vi "DeleteAction.vi"(8 "Error In":errorcluster, 9 "Analysis List":refnum<vi>, 10 "Analysis Step":i32[](listbox), 11 "CoordinatteEntry In":T1={"ProcessSetting"=[], "Project Name"="Parttern", "AnalysisSetting"=[], "Coord?"=FALSE, "OriginPointInfo"={"Output Original"=FALSE, "Origin Name"="", "Angle"=0.0, "Mode"=0, "OriginPoint"={"X"=0.0, "Y"=0.0}}, "CaliperSetting"=[], "CoordIndex"=[]} {"CaliperSetting"."CaliperEntry"."CaliperType" items=["Distance", "Mid Point", "Perpendicular Projection", "Lines Intersection", "Angle from Horizontal", "Angle from Vertical", "Angle Defined by 3 Points", "Angle Defined by 4 Points", "Bissecting Line", "Mid Line", "Center of Mass", "Area", "Line Fit", "Circle Fit", "Ellipse Fit"]; "OriginPointInfo"."Mode" items=["Horizontal Motion", "Vertical Motion", "Horizontal and Vertical Motion", "Horizontal. Vertical and Angular Motion"]; "AnalysisSetting"."ROI"."Contours"."Type" items=["No Selection", "Point", "Line", "Rectangle", "Oval", "Polygon", "Freehand Region", "Annulus", "Unused2", "Unused3", "Broken Line", "Freehand Line", "Rotated Rectangle"]}) -> (0 "Error Out":errorcluster, 3 "CoordinatteEntry Out":T1={"ProcessSetting"=[], "Project Name"="Parttern", "AnalysisSetting"=[], "Coord?"=FALSE, "OriginPointInfo"={"Output Original"=FALSE, "Origin Name"="", "Angle"=0.0, "Mode"=0, "OriginPoint"={"X"=0.0, "Y"=0.0}}, "CaliperSetting"=[], "CoordIndex"=[]} {"CaliperSetting"."CaliperEntry"."CaliperType" items=["Distance", "Mid Point", "Perpendicular Projection", "Lines Intersection", "Angle from Horizontal", "Angle from Vertical", "Angle Defined by 3 Points", "Angle Defined by 4 Points", "Bissecting Line", "Mid Line", "Center of Mass", "Area", "Line Fit", "Circle Fit", "Ellipse Fit"]; "OriginPointInfo"."Mode" items=["Horizontal Motion", "Vertical Motion", "Horizontal and Vertical Motion", "Horizontal. Vertical and Angular Motion"]; "AnalysisSetting"."ROI"."Contours"."Type" items=["No Selection", "Point", "Line", "Rectangle", "Oval", "Polygon", "Freehand Region", "Annulus", "Unused2", "Unused3", "Broken Line", "Freehand Line", "Rotated Rectangle"]})   [LabVIEW 2015]
uses:
  Control/CoordinatteEntry.ctl
  Process/Controls/Process_Setting.ctl
  Process/Controls/Process_Type.ctl
  Control/CoordinateAnalysisSetting.ctl
  Control/CoordinateCaliperSetting.ctl
  Caliper/Controls/CaliperDataEntry.ctl
  Caliper/Controls/CaliperType.ctl
  Caliper/Controls/SelectionListEntry.ctl
  Caliper/Controls/SelectionListEntryPointType.ctl
  Caliper/Controls/CaliperResult.ctl
  Analysis/Controls/Parttern Match/Analysis_PatternMatch_Parameter.ctl
panel:
  out "RootPath":path
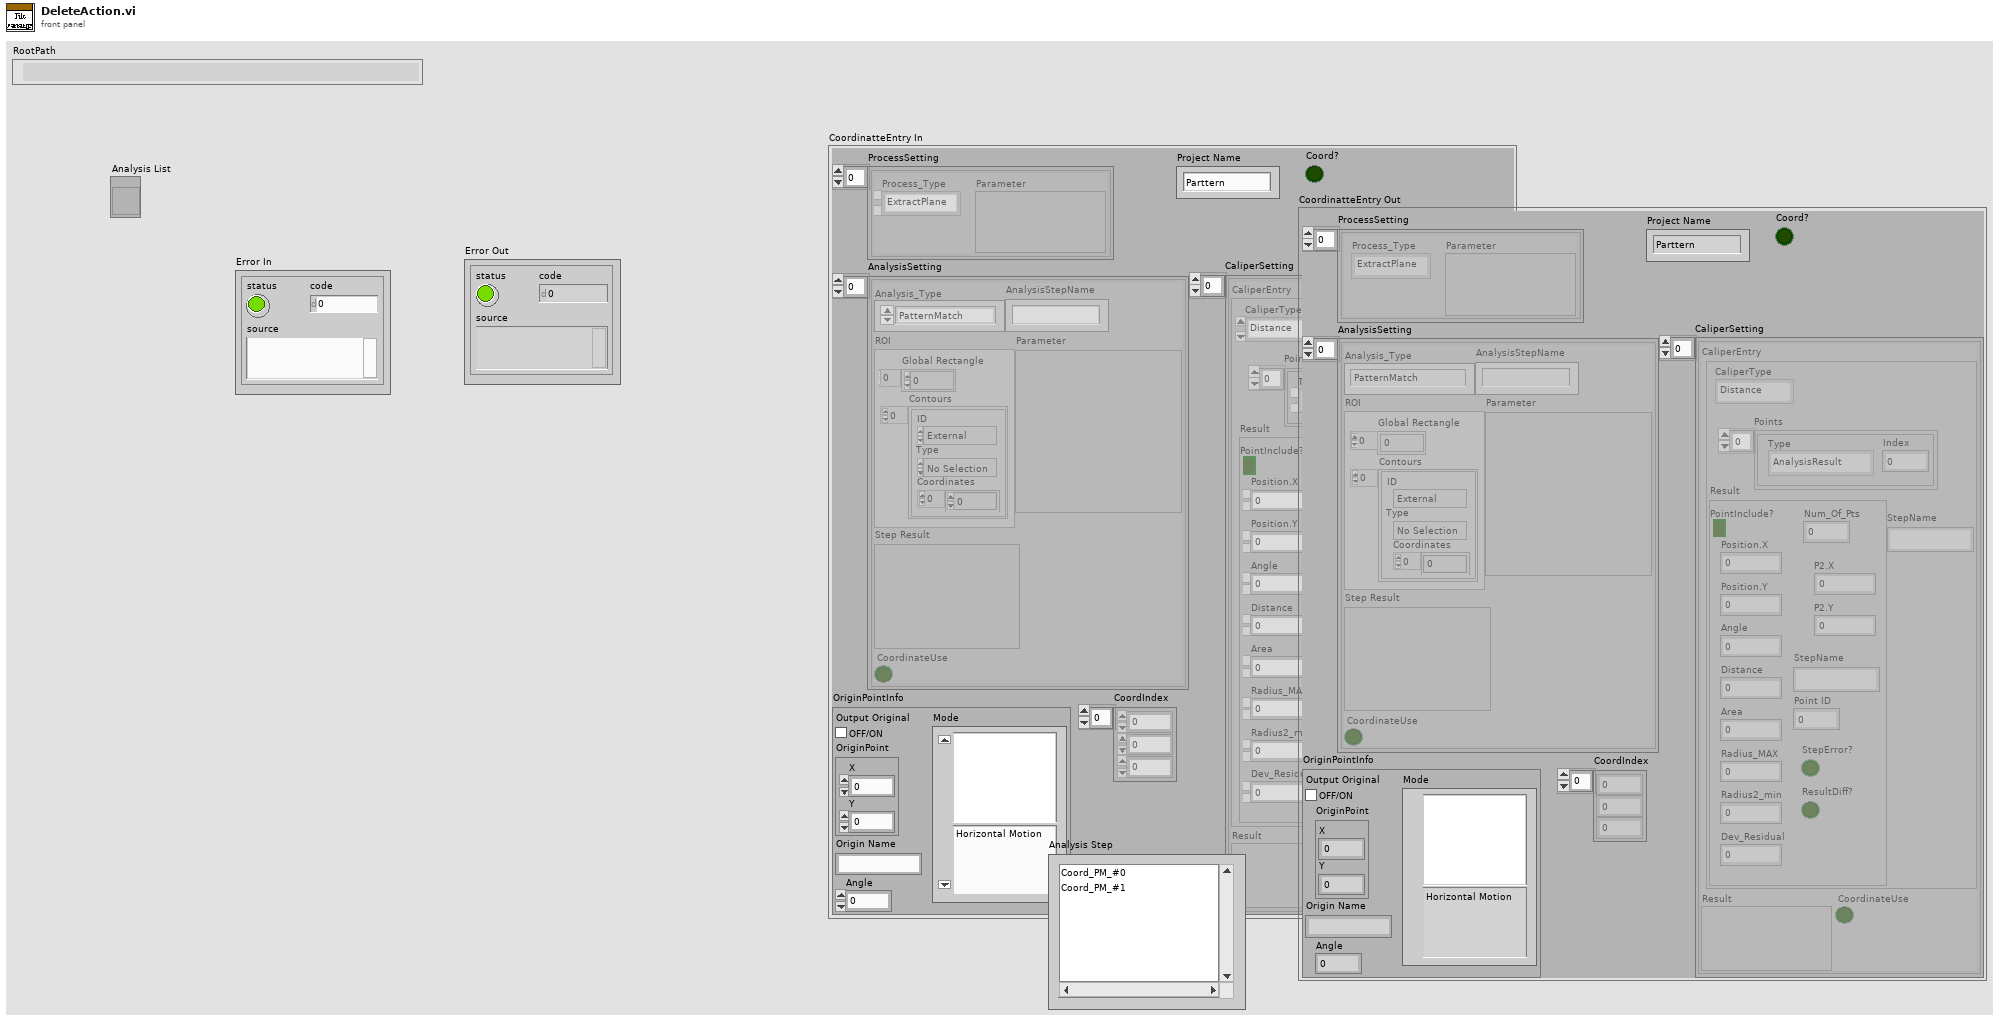
[diagram p1: front panel]
types:
  T1 = typedef "CoordinatteEntry.ctl" = cluster{"ProcessSetting":T2[], "Project Name":string, "AnalysisSetting":T4[], "Coord?":bool, "OriginPointInfo":cluster{"Output Original":bool, "Origin Name":string, "Angle":dbl, "Mode":u16, "OriginPoint":cluster{"X":dbl, "Y":dbl}}, "CaliperSetting":T6[], "CoordIndex":i32[]}
  T2 = typedef "Process_Setting.ctl" = cluster{"Process_Type":T3, "Parameter":variant}
  T3 = typedef "Process_Type.ctl" = enum16{"None", "ExtractPlane", "BinaryMono", "Operators", "GrayMorphology", "Filters", "Lookup Table", "Particle Filter", "Mask"}
  T4 = typedef "CoordinateAnalysisSetting.ctl" = cluster{"Analysis_Type":enum16{"PatternMatch", "Straight Edge"}, "ROI ":T5, "Parameter":variant, "Step Result":variant, "AnalysisStepName":string, "CoordinateUse":bool}
  T5 = typedef "ROI Descriptor" = cluster{"Global Rectangle":i32[], "Contours":cluster{"ID":enum32{"External", "Internal"}, "Type":u32, "Coordinates":i32[]}[]}
  T6 = typedef "CoordinateCaliperSetting.ctl" = cluster{"Result":variant, "CoordinateUse":bool, "CaliperEntry":T7}
  T7 = typedef "CaliperDataEntry.ctl" = cluster{"CaliperType":T8, "Points":T9[], "Result":T11, "StepName":string}
  T8 = typedef "CaliperType.ctl" = u32
  T9 = typedef "SelectionListEntry.ctl" = cluster{"Type":T10, "Index":i32}
  T10 = typedef "SelectionListEntryPointType.ctl" = enum16{"AnalysisResult", "CaliperResult"}
  T11 = typedef "CaliperResult.ctl" = cluster{"PointInclude?":bool, "Num_Of_Pts":u8, "Position.X":dbl, "Position.Y":dbl, "Angle":dbl, "Distance":dbl, "Area":dbl, "Radius_MAX":dbl, "Radius2_min":dbl, "Dev_Residual":dbl, "P2.X":dbl, "P2.Y":dbl, "StepName":string, "Point ID":u8, "StepError?":bool, "ResultDiff?":bool}
  T12 = enum32{"invalid app kind", "Development System", "Run Time System", "Student Edition", "Embedded LabVIEW", "Evaluation", "Custom"}
  T13 = typedef "Analysis_PatternMatch_Parameter.ctl" = cluster{"Algorithm":i32, "Match Parameters":cluster{"Number of Matches Requested":i32, "Minimum Match Score":sgl, "Angle Ranges":cluster{"Start Angle":sgl, "End Angle":sgl}[]}, "ROI Descriptor":T5, "Advanced Options":cluster{"Item":u16, "Value":dbl}[], "Template path":string, "XOffset":i32, "YOffset":i32}
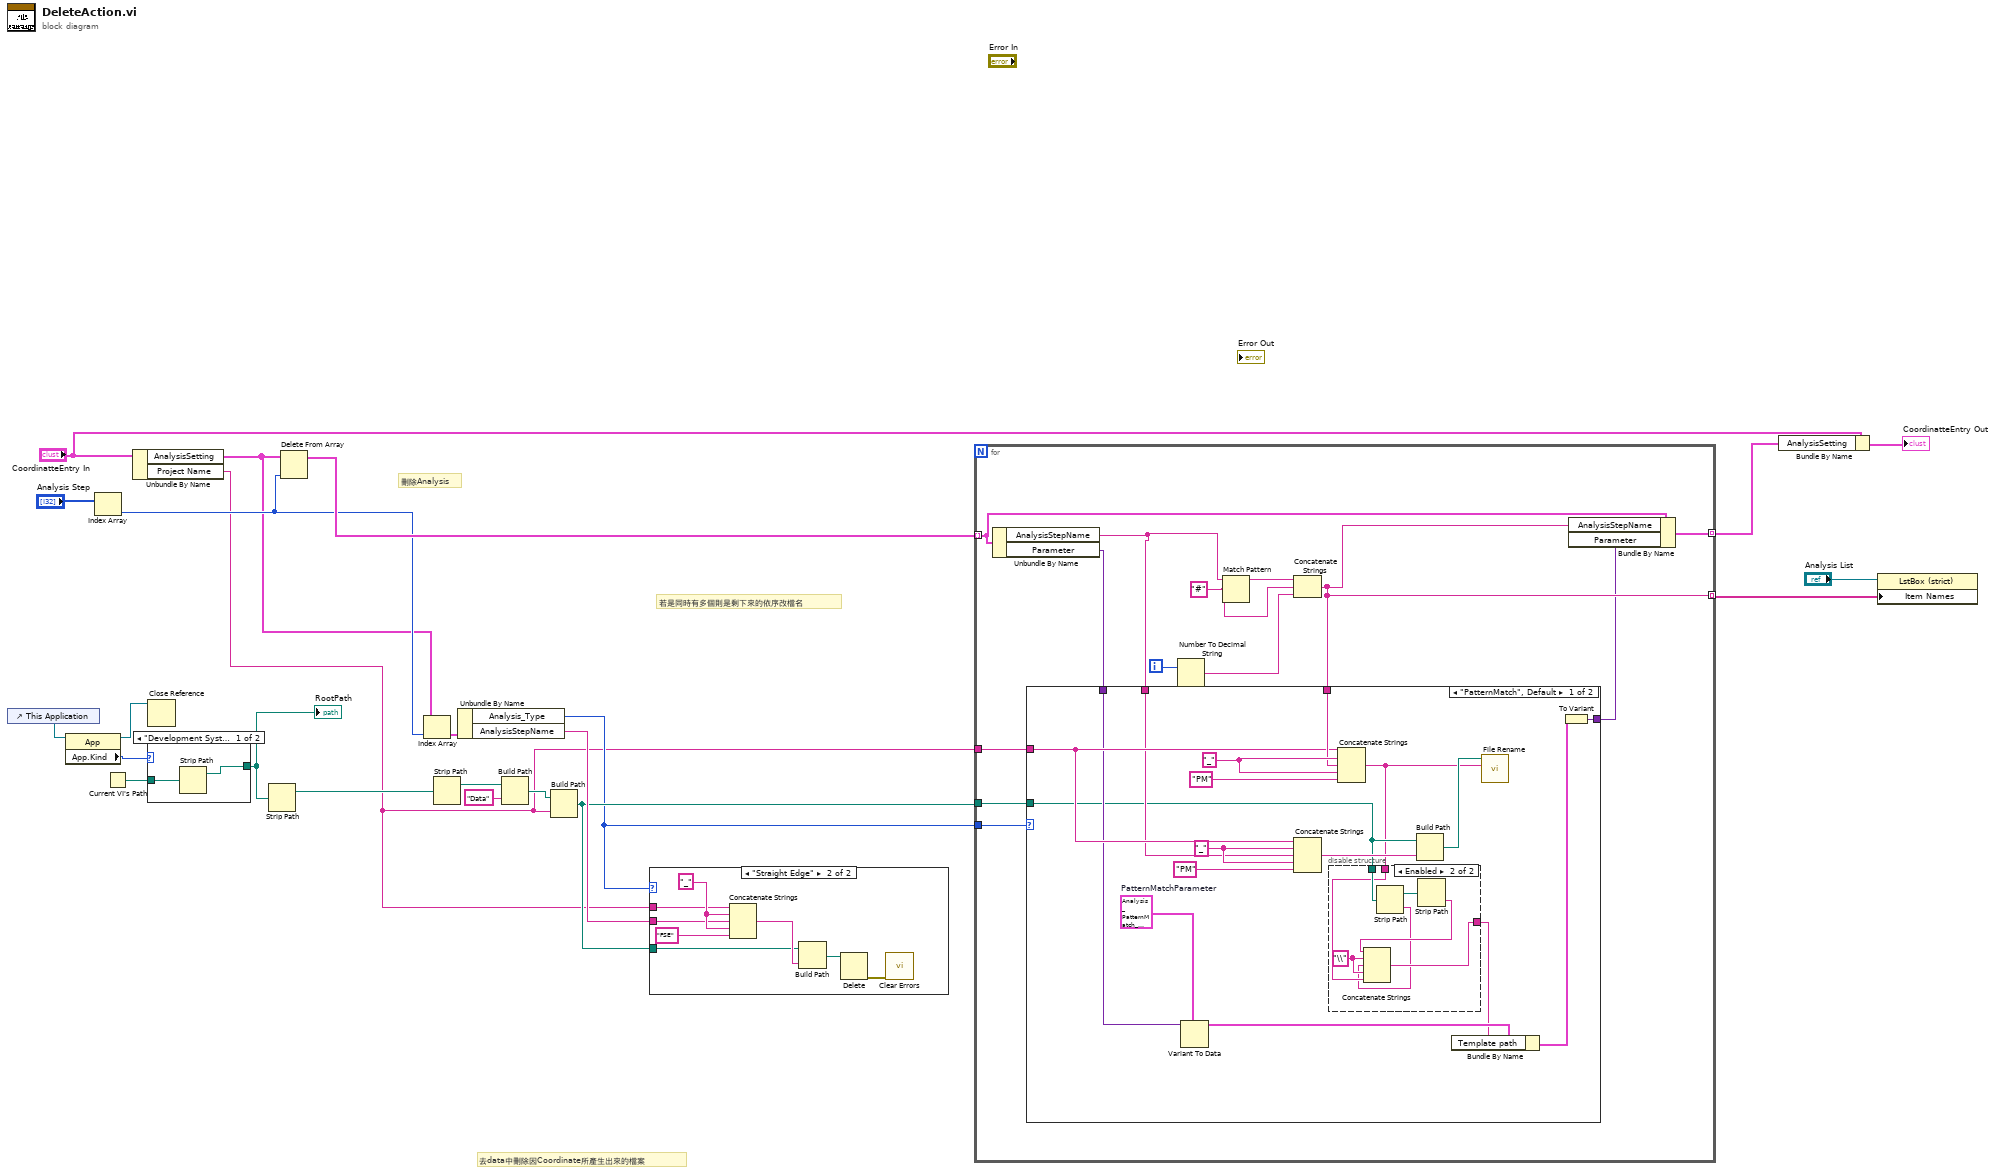
[diagram p0: block diagram]
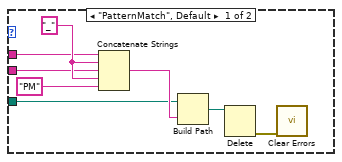
[diagram p2: hidden frame]
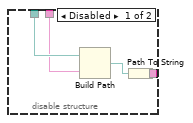
[diagram p3: hidden frame]
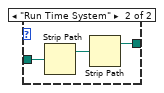
[diagram p5: hidden frame]
diagram:
  # "若是同時有多個則是剩下來的依序改檔名"
  # "去data中刪除因Coordinate所產生出來的檔案"
  # "刪除Analysis"
  n1 = control-ref of="This Application"() -> (w20:refnum<vi>)
  n2 = property class="App"(reference=w20) -> (reference out=w22:refnum<vi>, "App.Kind"=w21:T12)  [unwired: 1 in, 1 out]
  n3 = Index Array(array="Analysis Step") -> (element=w8:i32)  [unwired: 1 in]
  n4 = Current VI's Path() -> (path=w23:path)
  n5 = Unbundle By Name("CoordinatteEntry In") -> ("AnalysisSetting"=w6:T4[], "Project Name"=w1:string)
  n6 = case shown="\"Development System\", Default" w21 {
    tunnel: w23 -> [w25 w28]
    tunnel: [w24 w26] -> w19
    frame "Development System", Default {
      n7 = Strip Path(path=w25) -> (stripped path=w24:path)  [unwired: 1 out]
    }
    frame "Run Time System" {
      n8 = Strip Path(path=w28) -> (stripped path=w27:path)  [unwired: 1 out]
      n9 = Strip Path(path=w27) -> (stripped path=w26:path)  [unwired: 1 out]
    }
  }
  "RootPath" <- w19
  n10 = Close Reference(reference=w22) -> ()  [unwired: 1 in, 1 out]
  n11 = Strip Path(path=w19) -> (stripped path=w18:path)  [unwired: 1 out]
  n12 = Delete From Array "Delete From Array"(array=w6, index=w8) -> (array with subset deleted=w14:T4[])  [unwired: 1 in, 1 out]
  n13 = Index Array(array=w6, index=w8) -> (element=w7:T4)
  n14 = Strip Path(path=w18) -> (stripped path=w17:path)  [unwired: 1 out]
  n15 = Unbundle By Name(w7) -> ("Analysis_Type"=w2:enum16{"PatternMatch", "Straight Edge"}, "AnalysisStepName"=w4:string)
  n16 = Build Path(base path=w17, name or relative path="Data") -> (appended path=w15:path)
  n17 = Build Path(base path=w15, name or relative path=w1) -> (appended path=w3:path)
  n18 = case shown="\"Straight Edge\"" w2 {
    tunnel: w1 -> [w31 w39]
    tunnel: w4 -> [w30 w38]
    tunnel: w3 -> [w29 w37]
    frame "PatternMatch", Default {
      w35 = "_" ("string")
      n19 = Concatenate Strings(w31, w35, w30, w35, "PM" ("string")) -> (w33:string)
      n20 = Build Path(base path=w29, name or relative path=w33) -> (appended path=w32:path)
      n21 = Delete(path (use dialog)=w32) -> (error out=w34:errorcluster)  [unwired: 4 in, 2 out]
      n22 = call <vilib>:"Clear Errors.vi"("error in (no error)"=w34) -> ()  [unwired: 5 in, 2 out]
    }
    frame "Straight Edge" {
      w43 = "_" ("string")
      n23 = Concatenate Strings(w39, w43, w38, w43, "FSE" ("string")) -> (w41:string)
      n24 = Build Path(base path=w37, name or relative path=w41) -> (appended path=w40:path)
      n25 = Delete(path (use dialog)=w40) -> (error out=w42:errorcluster)  [unwired: 4 in, 2 out]
      n26 = call <vilib>:"Clear Errors.vi"("error in (no error)"=w42) -> ()  [unwired: 5 in, 2 out]
    }
  }
  n27 = for {
    tunnel: w14 -> [w53] mode=indexing
    tunnel: [w52] -> w12 mode=indexing
    tunnel: [w51] -> w9 mode=indexing
    tunnel: w1 -> [w50]
    tunnel: w3 -> [w48]
    tunnel: w2 -> [w47]
    i -> [w57]
    w55 = "#" ("regular expression")
    n28 = Unbundle By Name(w53) -> ("AnalysisStepName"=w49:string, "Parameter"=w46:variant)
    n29 = Number To Decimal String(number=w57) -> (decimal integer string=w54:string)  [unwired: 1 in]
    n30 = Match Pattern(string=w49, regular expression=w55) -> (before substring=w56:string)  [unwired: 1 in, 3 out]
    n31 = Concatenate Strings(w56, w55, w54) -> (w51:string)
    n32 = case shown="\"PatternMatch\", Default" w47 {
      tunnel: w51 -> [w72 _]
      tunnel: w50 -> [w69 _]
      tunnel: w49 -> [w68 _]
      tunnel: w48 -> [w62 _]
      tunnel: w46 -> [w65 w86]
      tunnel: [w59 w86] -> w45
      frame "PatternMatch", Default {
        w64 = T13 {"Algorithm"=2, "Match Parameters"={"Number of Matches Requested"=1, "Minimum Match Score"=750.0, "Angle Ranges"=[]}, "ROI Descriptor"={"Global Rectangle"=[], "Contours"=[]}, "Advanced Options"=[{"Item"=1, "Value"=1.0}, {"Item"=103, "Value"=1.0}], "Template path"="", "XOffset"=0, "YOffset"=0}  # PatternMatchParameter
        w70 = "_" ("string")
        w74 = "_" ("string")
        n33 = Variant To Data(type=w64, Variant=w65) -> (data=w63:T13)  [unwired: 1 in, 1 out]
        n34 = Concatenate Strings(w69, w70, w68, w70, "PM" ("string")) -> (w67:string)
        n35 = Concatenate Strings(w69, w74, w72, w74, "PM" ("string")) -> (w61:string)
        n36 = disable-structure shown="Enabled" {
          disable-tunnel: w62 -> [w78 w85]
          disable-tunnel: w61 -> [w77 w82]
          disable-tunnel: [w75 w81] -> w58
          frame Disabled {
            n37 = Build Path(base path=w78, name or relative path=w77) -> (appended path=w76:path)
            n38 = Path To String(path=w76) -> (string=w75:string)
          }
          frame Enabled {
            w83 = "\\" ("string")
            n39 = Strip Path(path=w85) -> (stripped path=w84:path, name=w79:string)
            n40 = Strip Path(path=w84) -> (name=w80:string)  [unwired: 1 out]
            n41 = Concatenate Strings(w80, w83, w79, w83, w82) -> (w81:string)
          }
        }
        n42 = Build Path(base path=w62, name or relative path=w67) -> (appended path=w66:path)
        n43 = Bundle By Name(cluster=w63, "Template path"=w58) -> (w60:T13)
        n44 = call "File Rename.vi"("name or relative path"=w61, "path"=w66) -> ()  [unwired: 10 in]
        n45 = To Variant(anything=w60) -> (Variant=w59:variant)
      }
      frame "Straight Edge" {
      }
    }
    n46 = Bundle By Name(cluster=w53, "AnalysisStepName"=w51, "Parameter"=w45) -> (w52:T4)
  }
  n47 = Bundle By Name(cluster="CoordinatteEntry In", "AnalysisSetting"=w12) -> (→"CoordinatteEntry Out":T1)
  n48 = property class="LstBox (strict)"(reference="Analysis List", "Item Names"=w9) -> ()  [unwired: 1 in, 2 out]
